vi "Set Wavelength.vi"(8 "error in":errorcluster, 10 "Wavelength (nm)":dbl, 11 "2936r in":refnum<class "2936r.lvclass">) -> (0 "error out":errorcluster, 3 "2936r out":refnum<class "2936r.lvclass">)   [LabVIEW 2018, in "2936r.lvlib" / "2936r.lvclass"]
uses:
  2936r.lvclass
  2936r.lvclass/2936r.ctl
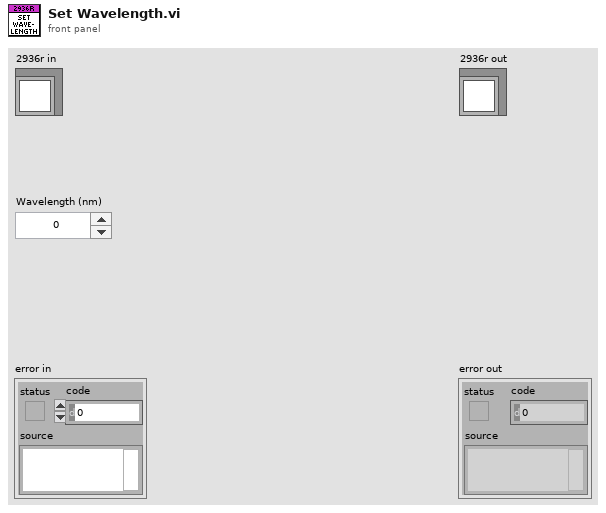
[diagram p1: front panel]
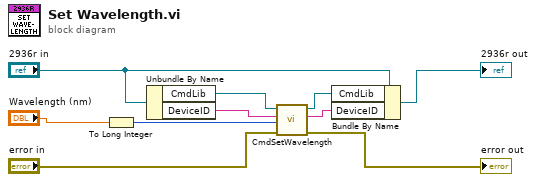
[diagram p0: block diagram]
diagram:
  n1 = To Long Integer(number="Wavelength (nm)") -> (32bit integer=w9:i32)
  n2 = Unbundle By Name("2936r in") -> ("CmdLib"=w8:refnum<k24>, "DeviceID"=w7:string)
  n3 = call <instrlib>:"CmdSetWavelength.vi"("error in (no error)"="error in", "Wavelength"=w9, "Device Key In"=w7, "CmdLib In"=w8) -> ("error out"=→"error out":errorcluster, "Device Key Out"=w5:string, "CmdLib Out"=w4:refnum<k24>)  [unwired: 4 in, 1 out]
  n4 = Bundle By Name(cluster="2936r in", "CmdLib"=w4, "DeviceID"=w5) -> (→"2936r out":refnum<class "2936r.lvclass">)
